vi "tcp_get_queue.vi"(7 "response?":bool=TRUE, 8 "error in":errorcluster, 10 "command queue":string[](array[string]), 11 "connection in":refnum<k5>) -> (0 "error out":errorcluster, 2 "output":cluster{string[], string[]}, 3 "connection out":refnum<k5>)   [LabVIEW 2025]
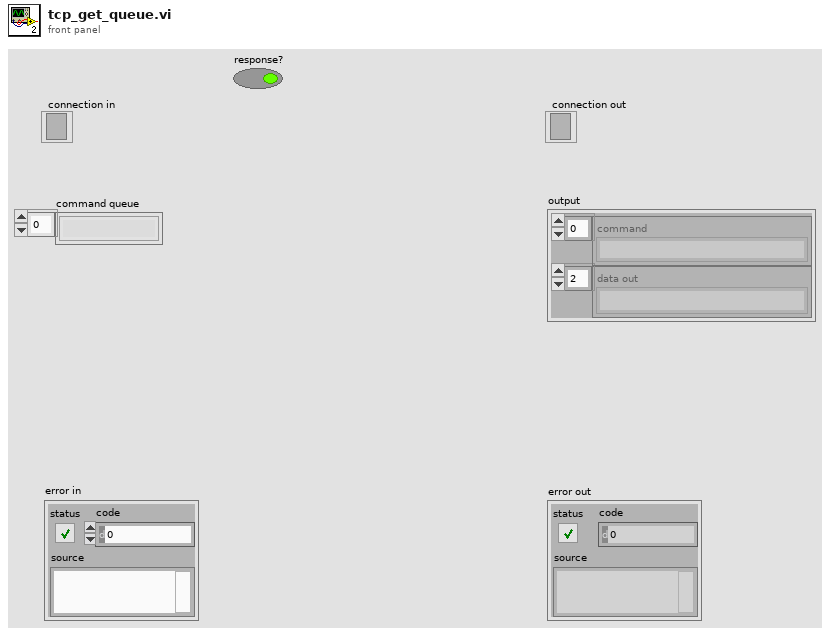
[diagram p1: front panel]
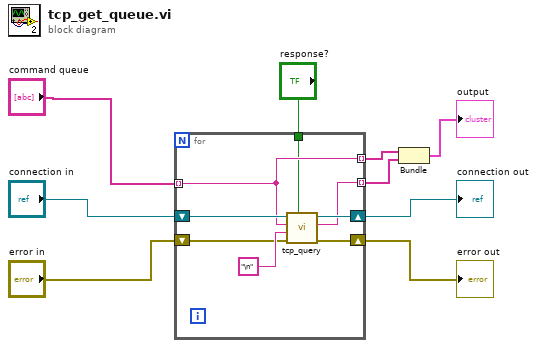
[diagram p0: block diagram]
diagram:
  n1 = for {
    tunnel: "command queue" -> [w13] mode=indexing
    tunnel: [w14] -> w6 mode=indexing
    tunnel: [w13] -> w5 mode=indexing
    tunnel: "response?" -> [w11]
    shift-right: [w15] -> w7
    shift-left: "error in" -> [w10]
    shift-right: [w16] -> w8
    shift-left: "connection in" -> [w17]
    n2 = call "tcp_query.vi"("response?"=w11, "error in (no error)"=w10, "Termination character"="\n", "Query String"=w13, "TCP Network Connection in"=w17) -> ("error out"=w15:errorcluster, "Message data out"=w14:string, "TCP Network Connection out"=w16:refnum<k5>)  [unwired: 4 in]
  }
  "connection out" <- w8
  "error out" <- w7
  n3 = Bundle(w5, w6) -> (→"output":cluster{string[], string[]})  [unwired: 1 in]
